vi "niScope Configure Trigger Runt.vi"(0 "instrument handle":refnum<k15>, 1 "polarity":T1=1 items=["Positive"=1, "Negative"=2, "Either"=3], 2 "trigger coupling":T3=1 items=["AC"=0, "DC"=1, "HF Reject"=3, "LF Reject"=4, "AC Plus HF Reject"=1001], 5 "trigger source":T2="0" caption="trigger source (Channel 0)", 7 "runt low threshold":dbl caption="low threshold" format="%^.3e", 9 "runt high threshold":dbl caption="high threshold" format="%^.3e", 11 "error in":errorcluster, 12 "trigger holdoff":dbl format="%.4f", 13 "trigger delay":dbl format="%.4f") -> (4 "instrument handle out":refnum<k15>, 15 "error out":errorcluster)   [LabVIEW 2020]
doc: "Configures common properties for runt triggering."
uses:
  niScope trigger coupling.ctl
  niScope trigger source.ctl
  niScope trigger polarity.ctl
  niScope_32.dll
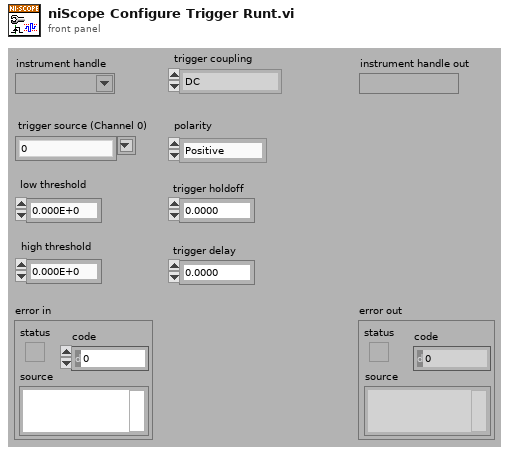
[diagram p1: front panel]
types:
  T1 = typedef "niScope trigger polarity.ctl" = i32
  T2 = typedef "niScope trigger source.ctl" = string
  T3 = typedef "niScope trigger coupling.ctl" = u16
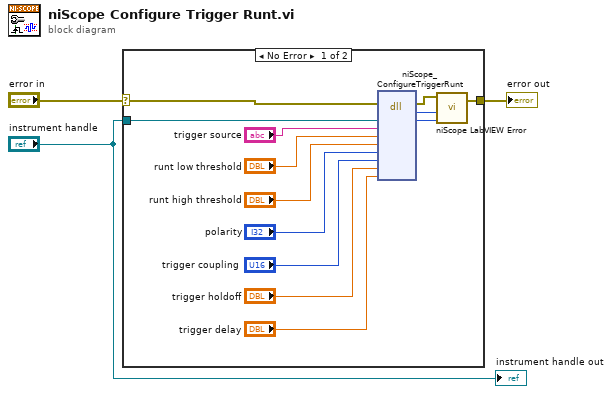
[diagram p0: block diagram]
diagram:
  n1 = case shown="No Error" "error in" {
    selector: "error in" -> [w5 w17]
    tunnel: [w13 w17] -> w3
    tunnel: "instrument handle" -> [w16 _]
    frame No Error {
      n2 = dll-call lib="niScope_*.*" fn="niScope_ConfigureTriggerRunt"(error in=w5, "instrument handle"=w16, "triggerSource"="trigger source", "runtLowThreshold"="runt low threshold", "runtHighThreshold"="runt high threshold", "runtPolarity"="polarity", "coupling"="trigger coupling", "holdoff"="trigger holdoff", "delay"="trigger delay") -> (error out=w4:errorcluster, "status"=w15:i32, "instrument handle"=w14:u32)  [unwired: 9 in, 1 out]
      n3 = call "niScope LabVIEW Error.vi"("instrument handle"=w14, "niScope error code (0)"=w15, "error in (no error)"=w4) -> ("error out"=w13:errorcluster)  [unwired: 2 in]
    }
    frame Error {
    }
  }
  "error out" <- w3
  "instrument handle out" <- "instrument handle"
